vi "LabviewDemo.vi"() -> ()   [LabVIEW 2021]
uses:
  vmmso/vmmso.lvlib
panel:
  out "IO Read Return":u32 format="%x"
  out "IO4":bool
  out "IO0":bool
  out "Is IO Ready":bool
  out "Is Data Ready？":bool
  in  "退出":bool
  in  "Start Capture":bool
  in  "Abort":bool
  out "Support Samples":u32[](array[numeric])
  out "InitDll Return":bool
  out "Device is OK?":bool
  out "FinishDll Return":i32
  out "Voltage Wave":dbl[](graph)
  out "ReadVoltageData Return":u32
  out "Capture Return":i32
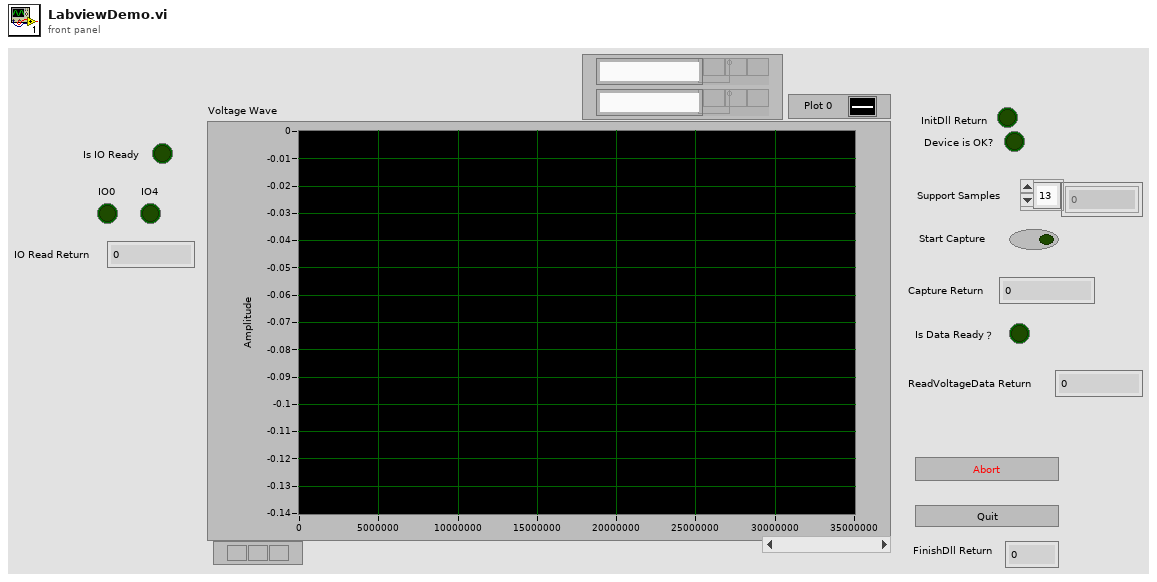
[diagram p1: front panel]
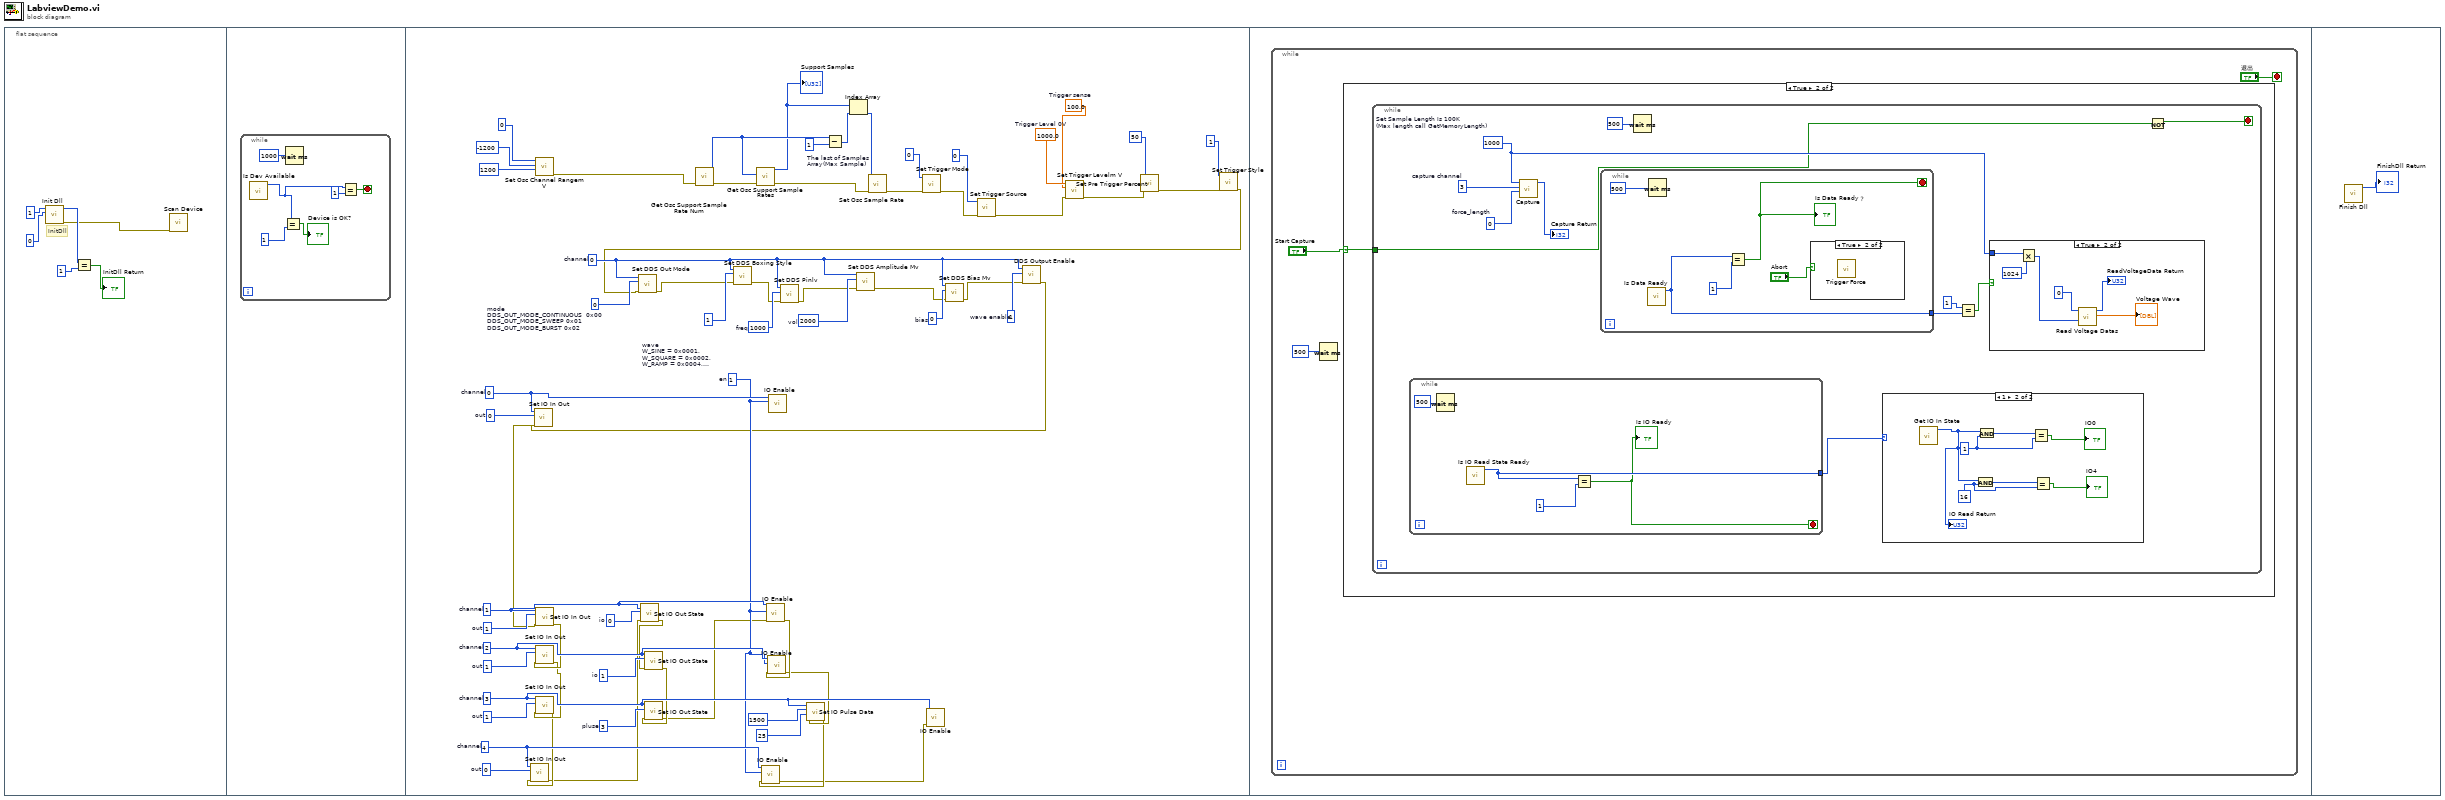
[diagram p0: block diagram]
diagram:
  n1 = flat-sequence {
    frame #0 {
      # "InitDll"
      n2 = call "Init Dll.vi"("en_hard_watchdog"=0 ("channel"), "en_log"=1 ("channel")) -> ("error out"=w1:errorcluster, "function return"=w2:i32)  [unwired: 8 in]
      n3 = Equal?(x=w2, y=1 ("channel")) -> (x = y?=→"InitDll Return":bool)
      n4 = call "Scan Device.vi"("error in (no error)"=w1) -> ()  [unwired: 9 in, 2 out]
    }
    frame #1 {
      n5 = while {
        stop <- w10 stop-if-true
        n6 = call "Is Dev Available.vi"() -> ("function return"=w9:i32)  [unwired: 10 in, 1 out]
        n7 = Equal?(x=w9, y=1 ("channel")) -> (x = y?=→"Device is OK?":bool)
        n8 = Wait (ms)(milliseconds to wait=u32 1000 ("等待时间（毫秒）")) -> ()  [unwired: 1 out]
        n9 = Equal?(x=w9, y=1) -> (x = y?=w10:bool)
      }
    }
    frame #2 {
      w42 = i8 0  # out
      w41 = i8 4  # channel
      w46 = i8 3  # pluse
      w47 = i8 1  # out
      w45 = i8 3  # channel
      w40 = i8 1  # en
      w51 = i8 0  # io
      w52 = i8 1  # io
      w53 = i8 1  # out
      w48 = i8 2  # channel
      w54 = i8 1  # out
      w49 = i8 1  # channel
      w55 = i8 0  # out
      w50 = i8 0  # channel
      w59 = sgl 100.0  # Trigger sense
      w60 = i8 0  # mode DDS_OUT_MODE_CONTINUOUS  0x00 DDS_OUT_MODE_SWEEP 0x01 DDS_OUT_MODE_BURST 0x02
      w62 = i8 1  # wave enable
      w64 = u32 0  # bias
      w63 = u32 2000  # vol
      w65 = u32 1000  # freq
      w66 = i8 1  # wave  W_SINE = 0x0001,  W_SQUARE = 0x0002,  W_RAMP = 0x0004,  W_PULSE = 0x0008,  W_NOISE = 0x0010,  W_DC = 0x0020,  W_ARB = 0x0040
      w61 = i8 0  # channel
      w75 = sgl 1000.0  # Trigger Level 0V
      n10 = call "Set Osc Channel Rangem V.vi"("maxmv"=1200 ("minmv"), "minmv"=-1200, "channel"=0) -> ("error out"=w39:errorcluster)  [unwired: 7 in, 1 out]
      n11 = call "Get Osc Support Sample Rate Num.vi"("error in (no error)"=w39) -> ("error out"=w38:errorcluster, "function return"=w71:i32)  [unwired: 9 in]
      n12 = call "Get Osc Support Sample Rates.vi"("error in (no error)"=w38, "maxnum"=w71) -> ("error out"=w37:errorcluster, "sample out"=w68:u32[])  [unwired: 7 in, 1 out]
      "Support Samples" <- w68
      n13 = call "IO Enable.vi"("enable"=w40, "channel"=w50) -> ()  [unwired: 9 in, 1 out]
      n14 = Subtract "The last of Samples Array(Max Sample)"(x=w71, y=1 ("front")) -> (x-y=w73:i32)
      n15 = Index Array(array=w68, index=w73) -> (element=w74:u32)
      n16 = call "Set Osc Sample Rate.vi"("error in (no error)"=w37, "sample"=w74) -> ("error out"=w36:errorcluster)  [unwired: 8 in, 1 out]
      n17 = call "Set Trigger Mode.vi"("error in (no error)"=w36, "mode"=0 ("front")) -> ("error out"=w35:errorcluster)  [unwired: 9 in]
      n18 = call "Set Trigger Source.vi"("error in (no error)"=w35, "source"=0 ("front")) -> ("error out"=w34:errorcluster)  [unwired: 9 in]
      n19 = call "Set Trigger Levelm V.vi"("error in (no error)"=w34, "sense_mv"=w59, "level_mv"=w75) -> ("error out"=w33:errorcluster)  [unwired: 8 in]
      n20 = call "Set Pre Trigger Percent.vi"("error in (no error)"=w33, "front"=50) -> ("error out"=w32:errorcluster)  [unwired: 9 in]
      n21 = call "Set Trigger Style.vi"("error in (no error)"=w32, "style"=u32 1) -> ("error out"=w31:errorcluster)  [unwired: 9 in]
      n22 = call "Set DDS Out Mode.vi"("error in (no error)"=w31, "out_mode"=w60, "channel_index"=w61) -> ("error out"=w30:errorcluster)  [unwired: 8 in]
      n23 = call "Set DDS Boxing Style.vi"("error in (no error)"=w30, "boxing"=w66, "channel_index"=w61) -> ("error out"=w29:errorcluster)  [unwired: 8 in]
      n24 = call "Set DDS Pinlv.vi"("error in (no error)"=w29, "pinlv"=w65, "channel_index"=w61) -> ("error out"=w28:errorcluster)  [unwired: 8 in]
      n25 = call "Set DDS Amplitude Mv.vi"("error in (no error)"=w28, "amplitdude"=w63, "channel_index"=w61) -> ("error out"=w27:errorcluster)  [unwired: 8 in]
      n26 = call "Set DDS Bias Mv.vi"("error in (no error)"=w27, "bias"=w64, "channel_index"=w61) -> ("error out"=w26:errorcluster)  [unwired: 8 in]
      n27 = call "DDS Output Enable.vi"("error in (no error)"=w26, "enable"=w62, "channel_index"=w61) -> ("error out"=w25:errorcluster)  [unwired: 8 in]
      n28 = call "Set IO In Out.vi"("error in (no error)"=w25, "inout"=w55, "channel"=w50) -> ("error out"=w24:errorcluster)  [unwired: 8 in]
      n29 = call "Set IO In Out.vi"("error in (no error)"=w24, "inout"=w54, "channel"=w49) -> ("error out"=w23:errorcluster)  [unwired: 8 in]
      n30 = call "Set IO In Out.vi"("error in (no error)"=w23, "inout"=w53, "channel"=w48) -> ("error out"=w22:errorcluster)  [unwired: 8 in]
      n31 = call "Set IO In Out.vi"("error in (no error)"=w22, "inout"=w47, "channel"=w45) -> ("error out"=w21:errorcluster)  [unwired: 8 in]
      n32 = call "Set IO In Out.vi"("error in (no error)"=w21, "inout"=w42, "channel"=w41) -> ("error out"=w20:errorcluster)  [unwired: 8 in]
      n33 = call "Set IO Out State.vi"("error in (no error)"=w20, "state"=w51, "channel"=w49) -> ("error out"=w19:errorcluster)  [unwired: 8 in]
      n34 = call "Set IO Out State.vi"("error in (no error)"=w19, "state"=w52, "channel"=w48) -> ("error out"=w18:errorcluster)  [unwired: 8 in]
      n35 = call "Set IO Out State.vi"("error in (no error)"=w18, "state"=w46, "channel"=w45) -> ("error out"=w17:errorcluster)  [unwired: 8 in]
      n36 = call "IO Enable.vi"("error in (no error)"=w17, "enable"=w40, "channel"=w49) -> ("error out"=w16:errorcluster)  [unwired: 8 in]
      n37 = call "IO Enable.vi"("error in (no error)"=w16, "enable"=w40, "channel"=w48) -> ("error out"=w15:errorcluster)  [unwired: 8 in]
      n38 = call "Set IO Pulse Data.vi"("error in (no error)"=w15, "duty"=25 ("minmv"), "hz"=1500 ("minmv"), "channel"=w45) -> ("error out"=w14:errorcluster)  [unwired: 7 in]
      n39 = call "IO Enable.vi"("error in (no error)"=w14, "enable"=w40, "channel"=w41) -> ("error out"=w13:errorcluster)  [unwired: 8 in]
      n40 = call "IO Enable.vi"("error in (no error)"=w13, "channel"=w45) -> ()  [unwired: 9 in, 1 out]
    }
    frame #3 {
      n41 = while {
        stop <- "退出" stop-if-true
        n42 = Wait (ms)(milliseconds to wait=u32 500 ("等待时间（毫秒）")) -> ()  [unwired: 1 out]
        n43 = case shown="True" "Start Capture" {
          selector: "Start Capture" -> [_ w80]
          frame False {
          }
          frame True {
            n44 = while {
              tunnel: w80 -> [w82]
              stop <- w83 stop-if-true
              w88 = i8 0  # force_length
              w86 = u32 1000  # Set Sample Length Is 100K (Max length call GetMemoryLength)
              w89 = i8 3  # capture channel
              n45 = while {
                tunnel: [w101] -> w81
                stop <- w99 stop-if-true
                n46 = Wait (ms)(milliseconds to wait=u32 500 ("等待时间（毫秒）")) -> ()  [unwired: 1 out]
                n47 = call "Is IO Read State Ready.vi"() -> ("function return"=w101:i32)  [unwired: 10 in, 1 out]
                n48 = Equal?(x=w101, y=1) -> (x = y?=w99:bool)
                "Is IO Ready" <- w99
              }
              n49 = call "Capture.vi"("force_length"=w88, "capture_channel"=w89, "length"=w86) -> ("function return"=→"Capture Return":i32)  [unwired: 7 in, 1 out]
              n50 = while {
                tunnel: [w111] -> w85
                stop <- w109 stop-if-true
                n51 = call "Is Data Ready.vi"() -> ("function return"=w111:i32)  [unwired: 10 in, 1 out]
                n52 = Wait (ms)(milliseconds to wait=u32 500 ("等待时间（毫秒）")) -> ()  [unwired: 1 out]
                n53 = Equal?(x=w111, y=1) -> (x = y?=w109:bool)
                "Is Data Ready？" <- w109
                n54 = case shown="True" "Abort" {
                  frame False {
                  }
                  frame True {
                    n55 = call "Trigger Force.vi"() -> ()  [unwired: 11 in, 1 out]
                  }
                }
              }
              n56 = Wait (ms)(milliseconds to wait=u32 500 ("等待时间（毫秒）")) -> ()  [unwired: 1 out]
              n57 = case shown="1" w81 {
                frame 0, Default {
                }
                frame 1 {
                  w97 = 16 ("front")
                  w94 = 1 ("front")
                  n58 = call "Get IO In State.vi"() -> ("function return"=w93:u32)  [unwired: 10 in, 1 out]
                  "IO Read Return" <- w93
                  n59 = And(x=w93, y=w97) -> (x .and. y?=w96:u32)
                  n60 = And(x=w93, y=w94) -> (x .and. y?=w92:u32)
                  n61 = Equal?(x=w92, y=w94) -> (x = y?=→"IO0":bool)
                  n62 = Equal?(x=w96, y=w97) -> (x = y?=→"IO4":bool)
                }
              }
              n63 = Equal?(x=1 ("y"), y=w85) -> (x = y?=w84:bool)
              n64 = case shown="True" w84 {
                tunnel: w86 -> [_ w105]
                frame False {
                }
                frame True {
                  n65 = Multiply(x=w105, y=1024) -> (x*y=w104:u32)
                  n66 = call "Read Voltage Datas.vi"("length"=w104, "channel"=i8 0) -> ("buffer out"=→"Voltage Wave":dbl[], "function return"=→"ReadVoltageData Return":u32)  [unwired: 7 in, 1 out]
                }
              }
              n67 = Not(x=w82) -> (.not. x?=w83:bool)
            }
          }
        }
      }
    }
    frame #4 {
      n68 = call "Finish Dll.vi"() -> ("function return"=→"FinishDll Return":i32)  [unwired: 10 in, 1 out]
    }
  }
